vi "FindSubpanels.SMOArray.vi"(6 "Append (F)":bool, 8 "error in":errorcluster, 10 "Subpanels":refnum<class "SMO.lvclass">[](array[class]), 11 "SMO.UI.MAUI in":refnum<class "SMO.UI.MAUI.lvclass">) -> (0 "error out":errorcluster, 3 "SMO.UI.MAUI out":refnum<class "SMO.UI.MAUI.lvclass">)   [LabVIEW 2019, in "SMO.UI.MAUI.lvclass"]
uses:
  SMO.UI.MAUI.lvclass
  <vilib>/JKI/JKI SMO/SMO/SMO.lvclass
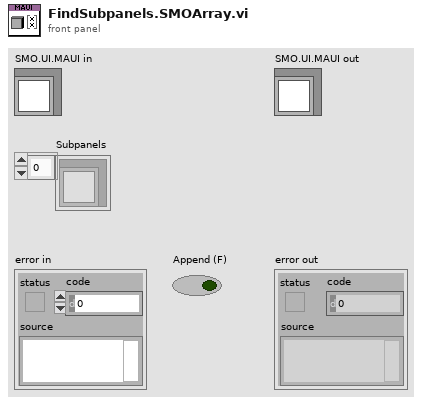
[diagram p1: front panel]
types:
  T1 = typedef "SMO.lvclass/SMOState --Enum.ctl" = enum16{"unknown", "Created", "Started", "Stopped"}
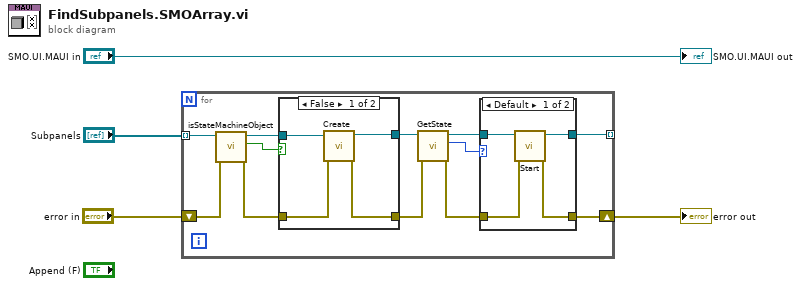
[diagram p0: block diagram]
diagram:
  n1 = for {
    tunnel: "Subpanels" -> [w16] mode=indexing
    shift-right: [w8] -> w1
    shift-left: "error in" -> [w7]
    tunnel: [w5] -> _ mode=indexing
    n2 = call <vilib>:"isStateMachineObject.vi"("error in (no error)"=w7, "SMO"=w16) -> ("error out"=w6:errorcluster, "is SMO?"=w15:bool, "SMO out"=w14:refnum<class "SMO.lvclass">)  [unwired: 7 in]
    n3 = case shown="False" w15 {
      tunnel: w14 -> [w26 w27]
      tunnel: [w25 w27] -> w13
      tunnel: w6 -> [w24 w28]
      tunnel: [w23 w28] -> w10
      frame False {
        n4 = call <vilib>:"Create.vi"("error in (no error)"=w24, "SMO"=w26) -> ("error out"=w23:errorcluster, "SMO out"=w25:refnum<class "SMO.lvclass">)  [unwired: 7 in, 1 out]
      }
      frame True {
      }
    }
    n5 = call <vilib>:"GetState.vi"("error in (no error)"=w10, "SMO"=w13) -> ("error out"=w9:errorcluster, "SMO State"=w11:T1, "SMO out"=w12:refnum<class "SMO.lvclass">)  [unwired: 7 in]
    n6 = case shown="Default" w11 {
      tunnel: w12 -> [w19 w22]
      tunnel: [w20 w22] -> w5
      tunnel: w9 -> [w17 w21]
      tunnel: [w18 w21] -> w8
      frame Default {
        n7 = call <vilib>:"Start.vi"("error in (no error)"=w17, "SMO"=w19) -> ("error out"=w18:errorcluster, "SMO out"=w20:refnum<class "SMO.lvclass">)  [unwired: 8 in]
      }
      frame "Started" {
      }
    }
  }
  "error out" <- w1
  "SMO.UI.MAUI out" <- "SMO.UI.MAUI in"
